vi "stopAllTasks.vi"(2 "error in":errorcluster, 3 "DAQ in":refnum<class "DAQ.lvclass">) -> (0 "error out":errorcluster, 1 "reference out":refnum<class "DAQ.lvclass">)   [LabVIEW 2017]
uses:
  classes/HardwareObjects/DAQ/DAQ.lvclass
  classes/HardwareObjects/DAQ/DAQ.lvclass/DAQ.ctl
  classes/HardwareObjects/DAQ/Read Master Counter Task.vi
  classes/HardwareObjects/DAQ/Read Galvo Counter Task.vi
  classes/HardwareObjects/DAQ/Read Galvo Analog Output Task.vi
  classes/HardwareObjects/DAQ/Read Camera Counter Task.vi
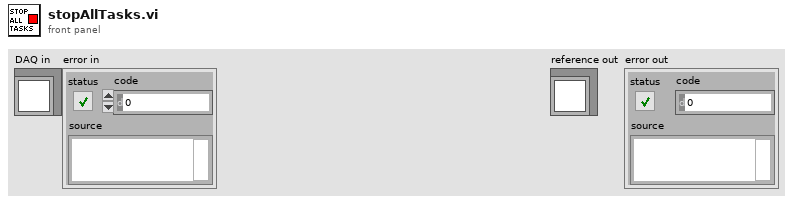
[diagram p1: front panel]
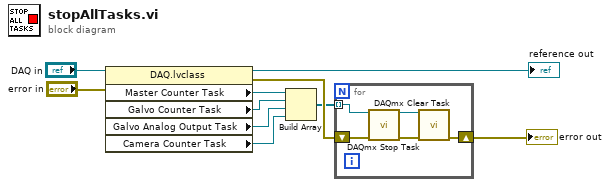
[diagram p0: block diagram]
diagram:
  n1 = property class="DAQ.lvclass"(reference="DAQ in", error in="error in") -> (reference out=→"reference out":refnum<class "DAQ.lvclass">, error out=w10:errorcluster, "Master Counter Task"=w9:refnum<k21>, "Galvo Counter Task"=w8:refnum<k21>, "Galvo Analog Output Task"=w7:refnum<k21>, "Camera Counter Task"=w6:refnum<k21>)
  n2 = Build Array(w9, w8, w7, w6) -> (w5:refnum<k21>[])
  n3 = for {
    shift-right: [w13] -> w1
    shift-left: w10 -> [w15]
    tunnel: w5 -> [w11] mode=indexing
    n4 = call <vilib>:"DAQmx Stop Task.vi"("task/channels in"=w11, "error in"=w15) -> ("task out"=w12:refnum<k21>, "error out"=w14:errorcluster)  [unwired: 12 in]
    n5 = call <vilib>:"DAQmx Clear Task.vi"("task in"=w12, "error in"=w14) -> ("error out"=w13:errorcluster)  [unwired: 13 in]
  }
  "error out" <- w1
